vi "init runtime test.vi"() -> ()   [LabVIEW 2013, in "Shared Library Module tests.lvlib"]
doc: "Platypus Framework 1.0.1.60\nNI Systems Engineering - National Instruments"
uses:
  Shared Library Module tests.lvlib
  <vilib>/NI/Tag Bus Module Framework/channel/channel classification.ctl
  configuration/Shared Library Module configuration.lvclass
  execution/Shared Library Module runtime.lvclass
  <vilib>/NI/Tag Bus/tag/tag descriptor.lvclass/tag descriptor.ctl
  <vilib>/NI/Tag Bus Module Framework/channel/TBM channel.lvclass/TBM channel.ctl
  <vilib>/NI/Tag Bus/tag/read tag name.vi
  <vilib>/NI/Tag Bus/tag/read data type.vi
  <vilib>/NI/Tag Bus Module Framework/channel/Read channel classification.vi
  <vilib>/NI/Tag Bus Module Framework/channel/TBM channel.lvclass
  <vilib>/NI/Tag Bus Module Framework/root configuration/TBM configuration.lvclass
  <vilib>/NI/Tag Bus/dictionary/data dictionary.lvclass
panel:
  out "tags found":bool
  out "no error":errorcluster
  out "expected execution settings":bool
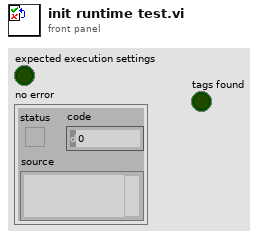
[diagram p1: front panel]
types:
  T1 = typedef "TBM channel.lvclass/channel classification.ctl" = enum16{"input data", "output data", "processing parameter", "processing result"}
  T2 = typedef "tag bus.lvlib/tag descriptor.lvclass/Data Type.ctl" = enum16{"Double", "Single", "I64", "I32", "I16", "I8", "U64", "U32", "U16", "U8", "Boolean", "String", "Array of Double", "Array of Single", "Array of I64", "Array of I32", "Array of I16", "Array of I8", "Array of U64", "Array of U32", "Array of U16", "Array of U8", "Array of Boolean", "Array of String"}
  T3 = typedef "TBM channel.lvclass/data tables.ctl" = cluster{"input data":T4, "processing parameter":T4, "processing result":T4, "output data":T4}
  T4 = typedef "tag bus.lvlib/dictionary table pair.ctl" = cluster{"data dictionary":refnum<class "data dictionary.lvclass">, "data table":T5}
  T5 = typedef "tag bus.lvlib/data table.lvlib/data table.ctl" = cluster{"Double":dbl[], "Single":sgl[], "I64":i64[], "I32":i32[], "I16":i16[], "I8":i8[], "U64":u64[], "U32":u32[], "U16":u16[], "U8":u8[], "Boolean":bool[], "String":string[], "Array of Double":cluster{"DBL Array":dbl[]}[], "Array of Single":cluster{"SGL Array":sgl[]}[], "Array of I64":cluster{"I64 Array":i64[]}[], "Array of I32":cluster{"I32 Array":i32[]}[], "Array of I16":cluster{"I16 Array":i16[]}[], "Array of I8":cluster{"I8 Array":i8[]}[], "Array of U64":cluster{"U64 Array":u64[]}[], "Array of U32":cluster{"U32 Array":u32[]}[], "Array of U16":cluster{"U16 Array":u16[]}[], "Array of U8":cluster{"U8 Array":u8[]}[], "Array of Boolean":cluster{"Boolean Array":bool[]}[], "Array of String":cluster{"String Array":string[]}[]}
  T6 = typedef "TBM module execution interface.lvclass/execution settings.ctl" = cluster{"reads inputs":bool, "processes data":bool, "writes outputs":bool}
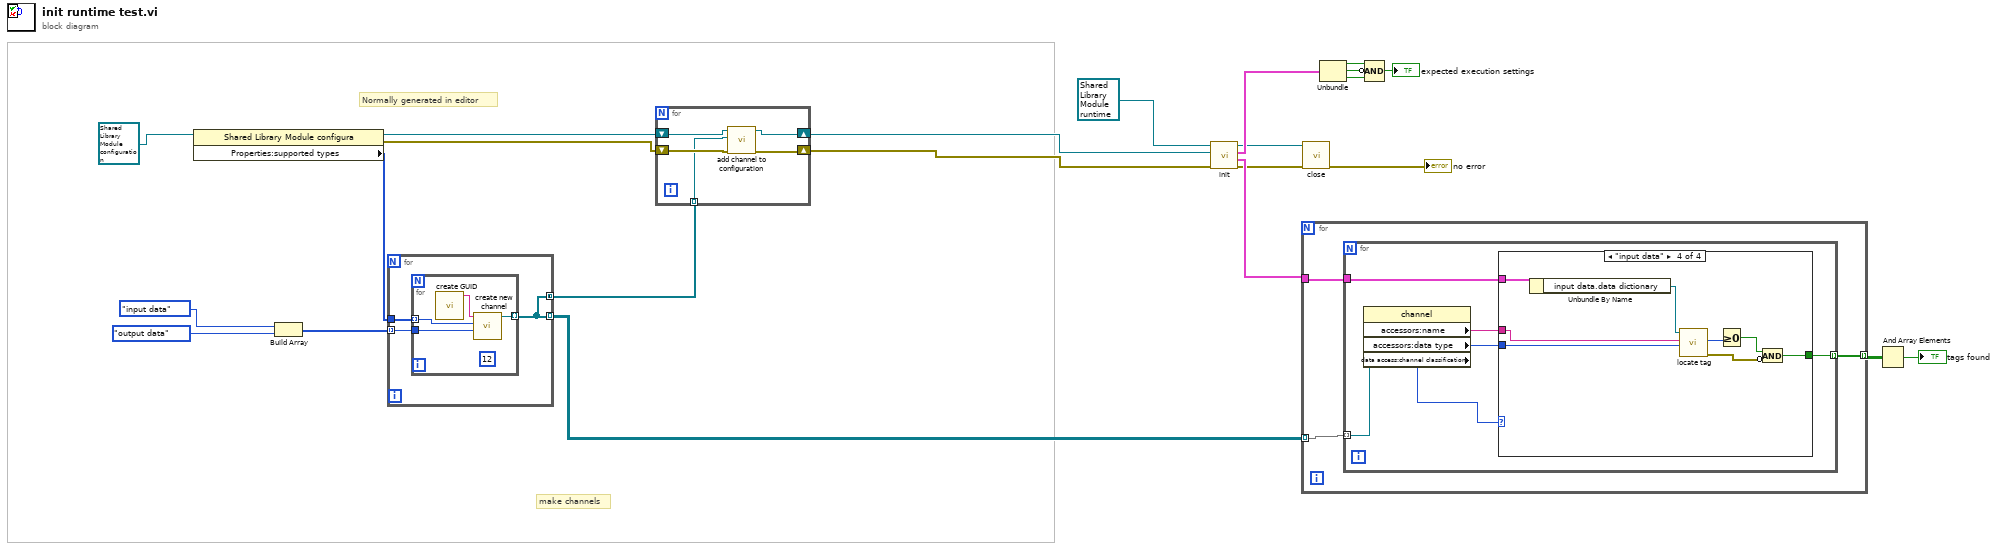
[diagram p0: block diagram]
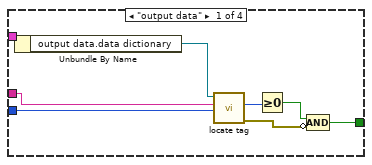
[diagram p2: hidden frame]
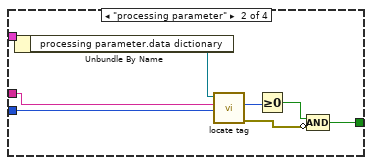
[diagram p3: hidden frame]
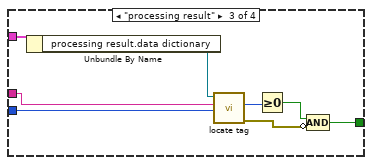
[diagram p4: hidden frame]
diagram:
  # "Normally generated in editor"
  # "make channels"
  n1 = property class="Shared Library Module configura"(reference=refnum<class "Shared Library Module configuration.lvclass"> refnum ("tag bus configurable plugin module configuration")) -> (reference out=w5:refnum<class "Shared Library Module configuration.lvclass">, error out=w3:errorcluster, "Properties:supported types"=w20:T2[])  [unwired: 1 in]
  n2 = Build Array(channel_classification."input data" ("channel classification"), channel_classification."output data" ("channel classification")) -> (w21:T1[])
  n3 = for {
    tunnel: w21 -> [w26] mode=indexing
    tunnel: [w24] -> w13 mode=indexing
    tunnel: w20 -> [w25]
    tunnel: [w24] -> w2 mode=concatenating
    n4 = for {
      tunnel: w26 -> [w29]
      tunnel: [w30] -> w24 mode=indexing
      tunnel: w25 -> [w28] mode=indexing
      (unwired) 12
      n5 = call <vilib>:"create GUID.vi"() -> ("uuid"=w27:string)  [unwired: 11 in]
      n6 = call <vilib>:"create new channel.vi"("channel classification"=w29, "data type"=w28, "channel name"=w27) -> ("channel"=w30:refnum<class "TBM channel.lvclass">)  [unwired: 8 in]
    }
  }
  n7 = for {
    shift-right: [w34] -> w4
    shift-left: w5 -> [w35]
    shift-right: [w33] -> w1
    shift-left: w3 -> [w32]
    tunnel: w2 -> [w31] mode=indexing
    n8 = call "add channel to configuration.vi"("error in"=w32, "TBM channel in"=w31, "Shared Library Module configuration in"=w35) -> ("error out"=w33:errorcluster, "Shared Library Module configuration out"=w34:refnum<class "Shared Library Module configuration.lvclass">)  [unwired: 7 in]
  }
  n9 = call-dynamic "init.vi"("error in"=w1, "TBM module configuration in"=w4, "Shared Library Module runtime in"=refnum<class "Shared Library Module runtime.lvclass"> refnum ("tag bus configurable plugin module")) -> ("error out"=w10:errorcluster, "data allocations"=w19:T3, "execution settings"=w18:T6, "Shared Library Module runtime out"=w9:refnum<class "Shared Library Module runtime.lvclass">)  [unwired: 5 in]
  n10 = for {
    tunnel: w19 -> [w38]
    tunnel: w13 -> [w37] mode=indexing
    tunnel: [w36] -> w12 mode=indexing
    n11 = for {
      tunnel: w38 -> [w42]
      tunnel: w37 -> [w44] mode=indexing
      tunnel: [w39] -> w36 mode=indexing
      n12 = property class="channel"(reference=w44) -> ("accessors:name"=w40:string, "accessors:data type"=w41:T2, "data access:channel classification"=w43:T1)  [unwired: 1 in, 2 out]
      n13 = case shown="\"input data\"" w43 {
        tunnel: w42 -> [w52 w60 w68 w76]
        tunnel: w41 -> [w50 w58 w66 w74]
        tunnel: w40 -> [w49 w57 w65 w73]
        tunnel: [w45 w53 w61 w69] -> w39
        frame "output data" {
          n14 = Unbundle By Name(w52) -> ("output data.data dictionary"=w51:refnum<class "data dictionary.lvclass">)
          n15 = call <vilib>:"locate tag.vi"("data type"=w50, "name"=w49, "data dictionary in"=w51) -> ("error out"=w46:errorcluster, "index"=w48:i32)  [unwired: 6 in, 1 out]
          n16 = Greater Or Equal To 0?(x=w48) -> (x >= 0?=w47:bool)
          n17 = Compound Arithmetic op=AND(w47, invert w46) -> (w45:bool)
        }
        frame "processing parameter" {
          n18 = Unbundle By Name(w60) -> ("processing parameter.data dictionary"=w59:refnum<class "data dictionary.lvclass">)
          n19 = call <vilib>:"locate tag.vi"("data type"=w58, "name"=w57, "data dictionary in"=w59) -> ("error out"=w54:errorcluster, "index"=w56:i32)  [unwired: 6 in, 1 out]
          n20 = Greater Or Equal To 0?(x=w56) -> (x >= 0?=w55:bool)
          n21 = Compound Arithmetic op=AND(w55, invert w54) -> (w53:bool)
        }
        frame "processing result" {
          n22 = Unbundle By Name(w68) -> ("processing result.data dictionary"=w67:refnum<class "data dictionary.lvclass">)
          n23 = call <vilib>:"locate tag.vi"("data type"=w66, "name"=w65, "data dictionary in"=w67) -> ("error out"=w62:errorcluster, "index"=w64:i32)  [unwired: 6 in, 1 out]
          n24 = Greater Or Equal To 0?(x=w64) -> (x >= 0?=w63:bool)
          n25 = Compound Arithmetic op=AND(w63, invert w62) -> (w61:bool)
        }
        frame "input data" {
          n26 = Unbundle By Name(w76) -> ("input data.data dictionary"=w75:refnum<class "data dictionary.lvclass">)
          n27 = call <vilib>:"locate tag.vi"("data type"=w74, "name"=w73, "data dictionary in"=w75) -> ("error out"=w70:errorcluster, "index"=w72:i32)  [unwired: 6 in, 1 out]
          n28 = Greater Or Equal To 0?(x=w72) -> (x >= 0?=w71:bool)
          n29 = Compound Arithmetic op=AND(w71, invert w70) -> (w69:bool)
        }
      }
    }
  }
  n30 = call-dynamic "close.vi"("error in"=w10, "Shared Library Module runtime in"=w9) -> ("error out"=→"no error":errorcluster)  [unwired: 9 in]
  n31 = Unbundle(w18) -> ("reads inputs"=w17:bool, "processes data"=w15:bool, "writes outputs"=w16:bool)
  n32 = Compound Arithmetic op=AND(w17, invert w15, w16) -> (→"expected execution settings":bool)
  n33 = And Array Elements(Boolean array=w12) -> (logical AND=→"tags found":bool)
